vi "Aero_Tunnel_Monitor_2.vi"() -> ()   [LabVIEW 2011]
uses:
  <vilib>/Platform/TimedLoop/XDataNode/timing_clust.ctl
  <vilib>/Platform/TimedLoop/XDataNode/nitl_modes.ctl
  <vilib>/Platform/TimedLoop/XDataNode/wakeup.ctl
  EnFlo_Software_SVN/trunk/EnFloSW/ADAM Client/Sub VIs/ADAM Controls/Update_scan_value.ctl
  <vilib>/Platform/TimedLoop/XDataNode/XDataNode.xnode
  <vilib>/Platform/TimedLoop/XDataNode/XDNodeRunTimeDep.lvlib
panel:
  in  "Stop":bool
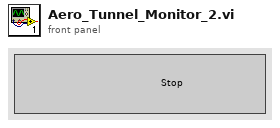
[diagram p1: front panel]
types:
  T1 = typedef "XDNodeRunTimeDep.lvlib/timing_clust.ctl" = cluster{"Expected End [f-1]":u64, "Actual End [f-1]":u64, "Finished Late? [f-1]":bool, "Expected End [i-1]":u64, "Actual End [i-1]":u64, "Finished Late? [i-1]":bool, "Expected Start [i]":u64, "Actual Start [i]":u64, "Expected Start [f]":u64, "Actual Start [f]":u64, "Source Name":string, "Structure Name":string, "Period":i64, "Deadline":i64, "Offset":i64, "Start":i64, "Priority":i32, "Timeout":i32, "Mode":T2, "Wakeup Reason":T3, "Error":errorcluster, "Source Type":string, "Secondary Source Type":string, "Global End Time":u64, "Global Start Time":u64, "Frame Duration":u64, "Iteration Duration":u64, "Assigned CPU":i32, "I/O Scan Engine Mode":u32}
  T2 = typedef "XDNodeRunTimeDep.lvlib/nitl_modes.ctl" = enum32{"No Change", "Process missed periods, maintain original phase", "Discard missed periods, maintain original phase", "Process missed periods, ignore original phase", "Discard missed periods, ignore original phase"}
  T3 = typedef "XDNodeRunTimeDep.lvlib/wakeup.ctl" = enum32{"Normal", "Aborted", "Asynchronous wakeup", "Timing source error", "Timed loop error", "Timeout"}
  T4 = typedef "Update_scan_value.ctl" = cluster{"Channel Name":string, "New Value":dbl}
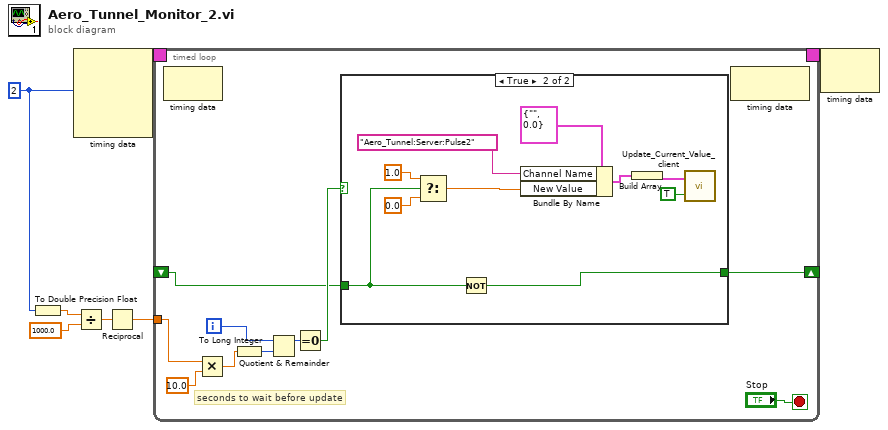
[diagram p0: block diagram]
diagram:
  w5 = i64 2 ("Period")
  n1 = To Double Precision Float(number=w5) -> (double precision float=w4:dbl)
  n2 = node-c288(w5) -> (w7:T1)  [unwired: 3 in]
  n3 = Divide(x=w4, y=1000.0) -> (x/y=w2:dbl)
  n4 = Reciprocal(x=w2) -> (1/x=w1:dbl)
  n5 = timed-loop {
    timing: w7 -> [_]
    timing-out: [_] -> w6
    shift-right: [w10] -> _
    shift-left: _ -> [w11]
    tunnel: w1 -> [w16]
    i -> [w14]
    stop <- "Stop" stop-if-true
    # "seconds to wait before update"
    n6 = node-c288() -> ()  [unwired: 1 in, 1 out]
    n7 = Multiply(x=w16, y=10.0) -> (x*y=w15:dbl)
    n8 = To Long Integer(number=w15) -> (32bit integer=w13:i32)
    n9 = Quotient & Remainder(x=w14, y=w13) -> (x-y*floor(x/y)=w9:i32)  [unwired: 1 out]
    n10 = Equal To 0?(x=w9) -> (x = 0?=w12:bool)
    n11 = case shown="True" w12 {
      tunnel: w11 -> [w18 w19]
      tunnel: [w18 w23] -> w10
      frame False {
      }
      frame True {
        n12 = Select(t=1.0, s=w19, f=0.0) -> (s? t:f=w20:dbl)
        n13 = Not(x=w19) -> (.not. x?=w23:bool)
        n14 = Bundle By Name(cluster=T4 {"Channel Name"="", "New Value"=0.0} ("Update Scan Value Cluster"), "Channel Name"="Aero_Tunnel:Server:Pulse2", "New Value"=w20) -> (w27:T4)
        n15 = Build Array(w27) -> (w26:T4[])
        n16 = call "Update_Current_Value_client.vi"("Don't Bother with check?"=TRUE, "Update array in"=w26) -> ()
      }
    }
    n17 = node-c288() -> ()  [unwired: 1 in, 1 out]
  }
  n18 = node-c288(w6) -> ()  [unwired: 1 out]
